vi "Get Oven Temperature.vi"(8 "error in (no error)":errorcluster, 11 "Owlstone GEN-SYS in":refnum<class "Owlstone GEN-SYS.lvclass">) -> (0 "error out":errorcluster, 1 "Temperature Setpoint":sgl, 2 "Temperature Value":sgl, 3 "Owlstone GEN-SYS out":refnum<class "Owlstone GEN-SYS.lvclass">)   [LabVIEW 2011, in "Owlstone GEN-SYS.lvclass"]
uses:
  Owlstone GEN-SYS.lvclass
  Owlstone GEN-SYS.lvclass/Owlstone GEN-SYS.ctl
  <instrlib>/Eurotherm 32xx Series/Eurotherm 32xx Series.lvlib
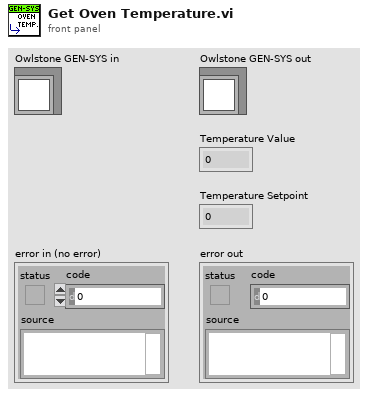
[diagram p1: front panel]
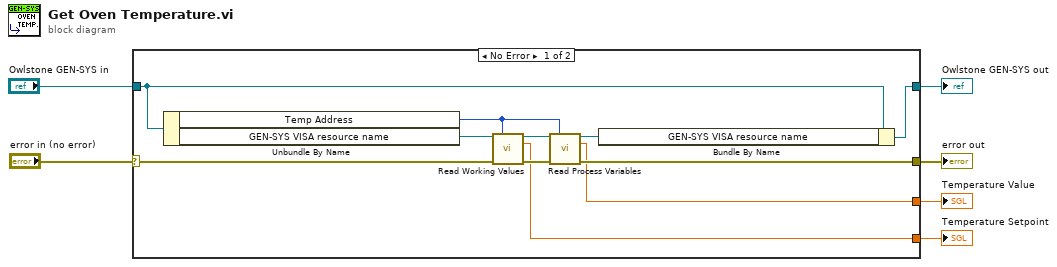
[diagram p0: block diagram]
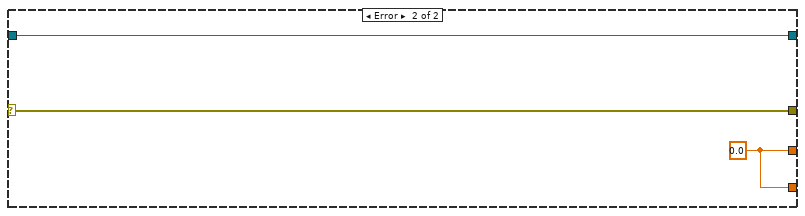
[diagram p2: hidden frame]
diagram:
  n1 = case shown="No Error" "error in (no error)" {
    selector: "error in (no error)" -> [w7 w19]
    tunnel: [w17 w20] -> w6
    tunnel: [w15 w19] -> w5
    tunnel: [w12 w18] -> w4
    tunnel: [w11 w18] -> w3
    tunnel: "Owlstone GEN-SYS in" -> [w10 w20]
    frame No Error {
      n2 = Unbundle By Name(w10) -> ("Temp Address"=w9:u8, "GEN-SYS VISA resource name"=w8:refnum<visa-resource-name>)
      n3 = call <instrlib>:"Read Working Values.vi"("VISA resource name"=w8, "Unit Address (1)"=w9, "error in (no error)"=w7) -> ("VISA resource name out"=w13:refnum<visa-resource-name>, "Working Setpoint (0)"=w12:sgl, "error out"=w14:errorcluster)  [unwired: 9 in, 1 out]
      n4 = call <instrlib>:"Read Process Variables.vi"("VISA resource name"=w13, "Unit Address (1)"=w9, "error in (no error)"=w14) -> ("VISA resource name out"=w16:refnum<visa-resource-name>, "Process Value"=w11:sgl, "error out"=w15:errorcluster)  [unwired: 9 in, 1 out]
      n5 = Bundle By Name(cluster=w10, "GEN-SYS VISA resource name"=w16) -> (w17:refnum<class "Owlstone GEN-SYS.lvclass">)
    }
    frame Error {
      w18 = sgl 0.0 ("Process Value")
    }
  }
  "Owlstone GEN-SYS out" <- w6
  "error out" <- w5
  "Temperature Setpoint" <- w4
  "Temperature Value" <- w3
